vi "Float Precision.vi"(8 "Enum":enum16{"Set", "Get"}(ring), 11 "Precision":string) -> (3 "Format String":string)   [LabVIEW 2017, in "API String Arguments Support.lvlib"]
uses:
  API String Arguments Support.lvlib
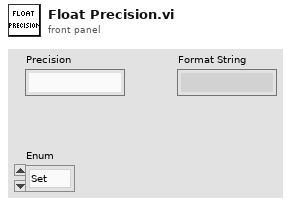
[diagram p1: front panel]
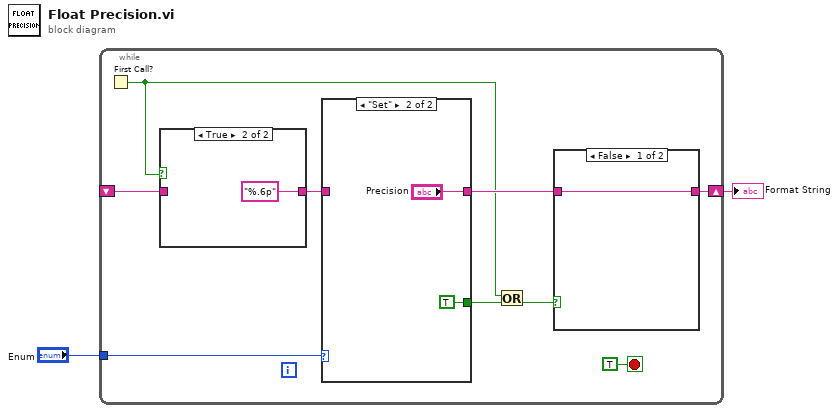
[diagram p0: block diagram]
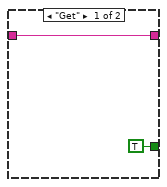
[diagram p3: hidden frame]
diagram:
  n1 = while {
    tunnel: "Enum" -> [w10]
    shift-right: [w7] -> w1
    shift-left: _ -> [w3]
    stop <- TRUE stop-if-true
    n2 = First Call?() -> (First Call?: T/F=w5:bool)
    n3 = case shown="True" w5 {
      tunnel: [w12 "%.6p" ("format string")] -> w4
      tunnel: w3 -> [w12 _]
      frame False {
      }
      frame True {
      }
    }
    n4 = case shown="\"Set\"" w10 {
      tunnel: [TRUE TRUE] -> w9
      tunnel: w4 -> [w14 _]
      tunnel: [w14 "Precision"] -> w6
      frame "Get" {
      }
      frame "Set" {
      }
    }
    n5 = Or(x=w5, y=w9) -> (x .or. y?=w8:bool)
    n6 = case shown="False" w8 {
      tunnel: [w18 w19] -> w7
      tunnel: w6 -> [w18 w19]
      frame False {
      }
      frame True {
      }
    }
  }
  "Format String" <- w1
